vi "Main On Compile Action VI_Parse DMA Block Prop.vi"(5 "Decimation FIFO Index":i32, 8 "error in (no error)":errorcluster, 9 "FIFO indexes":i32[](array[numeric])=[1, 2, 3, 4, 5], 10 "Block Address":u32[](array[numeric])=[0, 2, 2, 0, 3], 11 "Relative Address in Block":u32[](array[numeric])=[0, 0, 1, 5, 5]) -> (0 "error out":errorcluster, 2 "Block descriptor":T1, 3 "max block size":u32)   [LabVIEW 2019, in "RefMem DMA System Explorer.lvlib"]
uses:
  RefMem DMA System Explorer.lvlib
  Shared/Block descriptor.ctl
  Shared/RefMem DMA Shared.lvlib
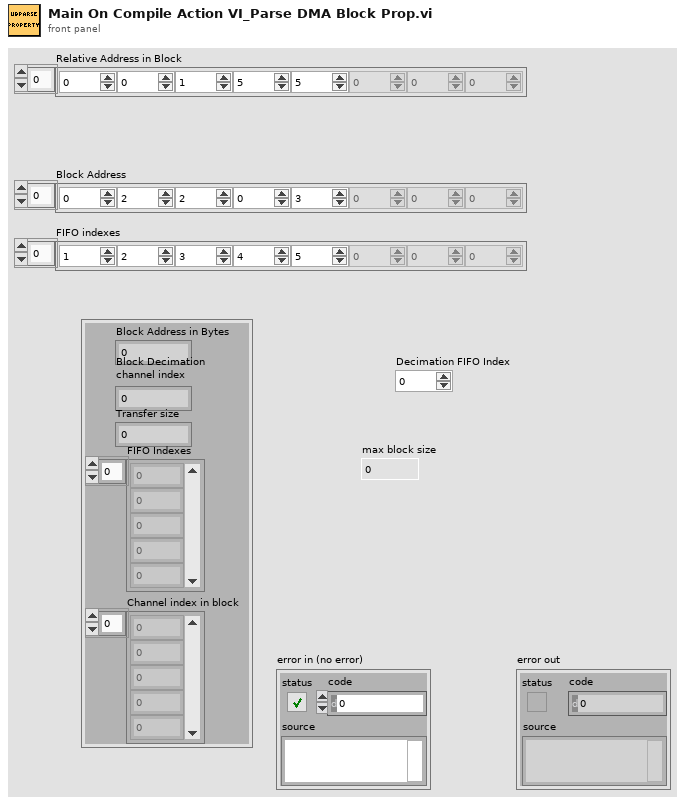
[diagram p1: front panel]
types:
  T1 = typedef "RefMem DMA Shared.lvlib/Block descriptor.ctl" = cluster{"Block Address in Bytes":u32, "Block Decimation \nchannel index":i32, "Transfer size":u32, "FIFO Indexes":i32[], "Channel index in block":i32[]}
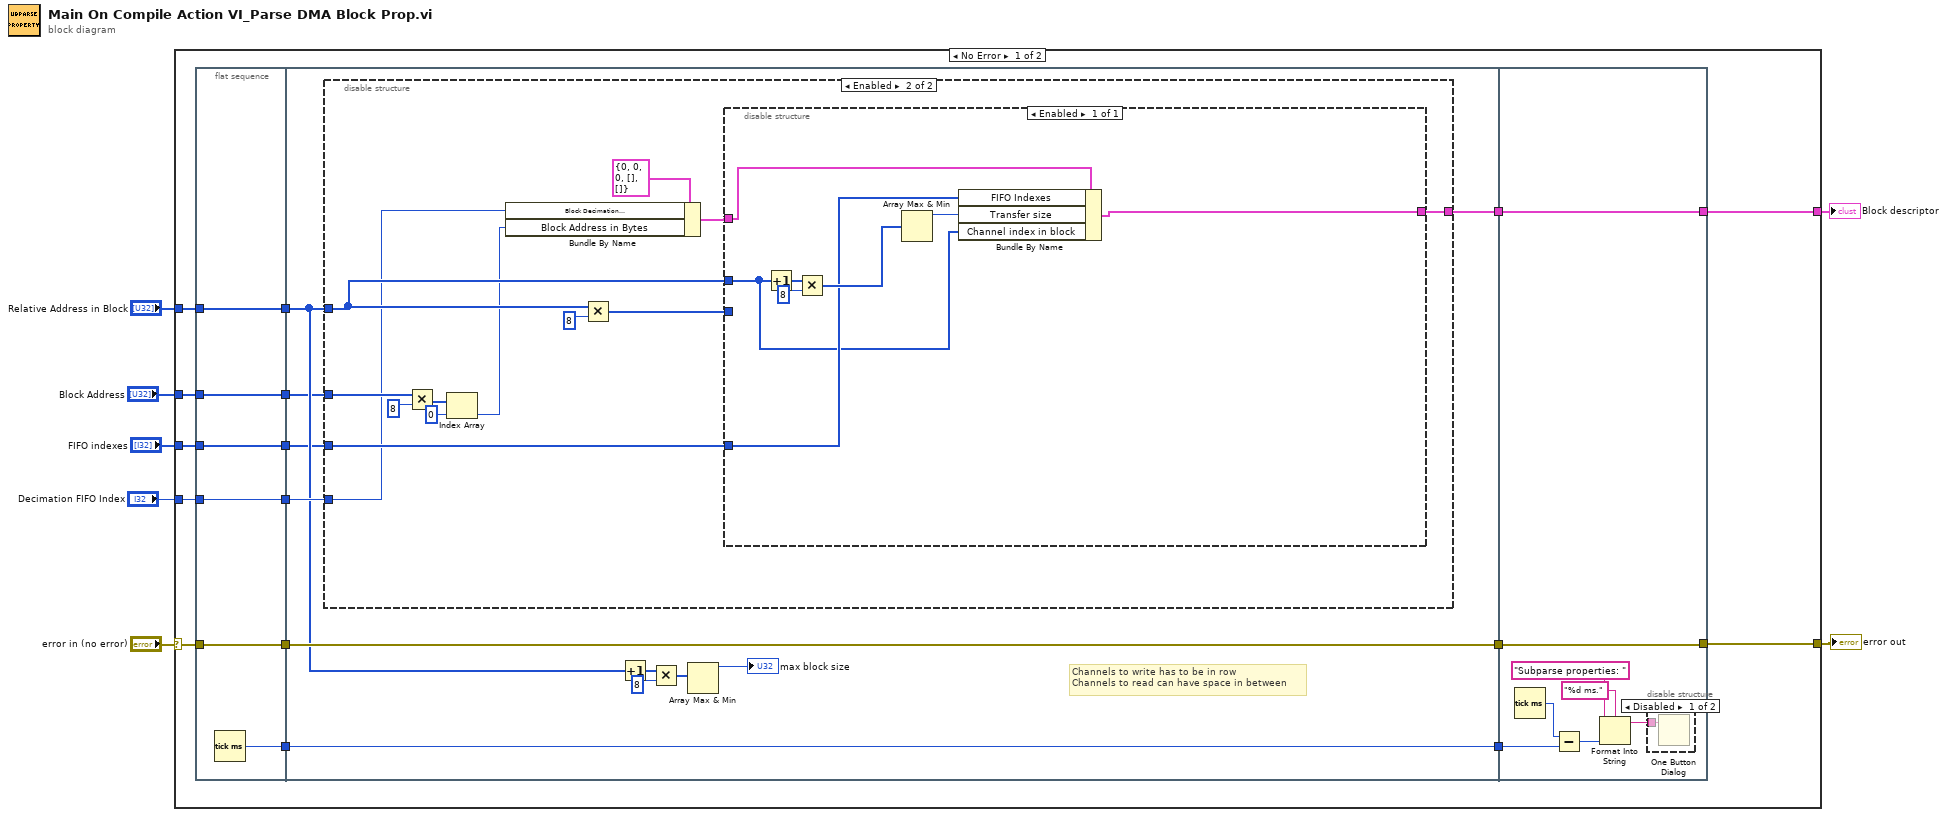
[diagram p0: block diagram]
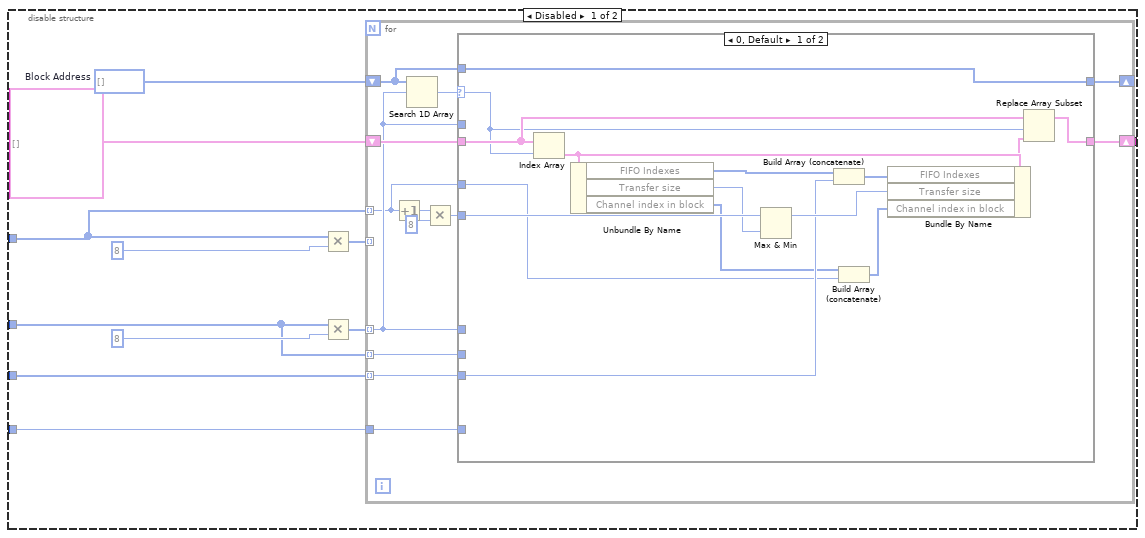
[diagram p2: hidden frame]
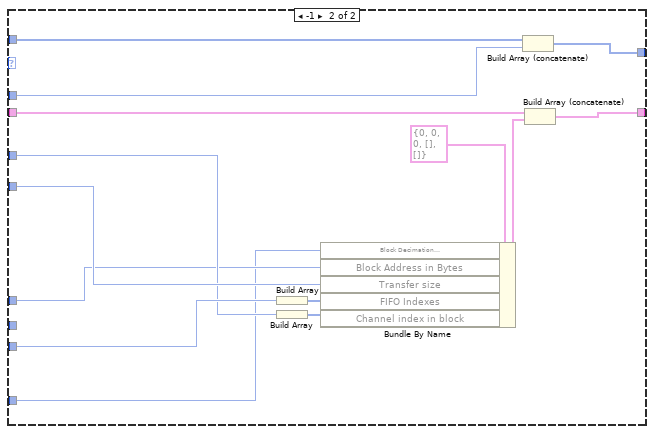
[diagram p3: hidden frame]
diagram:
  n1 = case shown="No Error" "error in (no error)" {
    selector: "error in (no error)" -> [w20 w124]
    tunnel: [w21 _] -> w7
    tunnel: [w18 w124] -> w5
    tunnel: "Decimation FIFO Index" -> [w17 _]
    tunnel: "Relative Address in Block" -> [w16 _]
    tunnel: "Block Address" -> [w15 _]
    tunnel: "FIFO indexes" -> [w14 _]
    frame No Error {
      n2 = flat-sequence {
        tunnel: w14 -> [w25]
        tunnel: w15 -> [w26]
        tunnel: w16 -> [w27]
        tunnel: w17 -> [w28]
        tunnel: w20 -> [w29]
        tunnel: [w29] -> w13
        tunnel: [w28] -> w12
        tunnel: [w27] -> w11
        tunnel: [w26] -> w10
        tunnel: [w25] -> w9
        tunnel: [w24] -> w8
        tunnel: [w40] -> w23
        tunnel: [w30] -> w22
        tunnel: [w35] -> w19
        tunnel: w13 -> [w35]
        tunnel: w12 -> [w34]
        tunnel: w11 -> [w33]
        tunnel: w10 -> [w32]
        tunnel: w9 -> [w31]
        tunnel: w8 -> [w30]
        tunnel: [w122] -> w21
        tunnel: w23 -> [w122]
        tunnel: w22 -> [w120]
        tunnel: w19 -> [w115]
        tunnel: [w115] -> w18
        frame #0 {
          n3 = Tick Count (ms)() -> (millisecond timer value=w24:u32)
        }
        frame #1 {
          # "Channels to write has to be in row\nChannels to read can have space in between"
          n4 = disable-structure shown="Enabled" {
            disable-tunnel: [w49 w106] -> w40
            disable-tunnel: w34 -> [w44 w98]
            disable-tunnel: w33 -> [w43 w102]
            disable-tunnel: w32 -> [w42 w101]
            disable-tunnel: w31 -> [w41 w100]
            frame Disabled {
              w51 = u32[] []  # Block Address
              n5 = Multiply(x=w43, y=u32 8) -> (x*y=w47:u32[])
              n6 = Multiply(x=w42, y=u32 8) -> (x*y=w45:u32[])
              n7 = for {
                tunnel: w45 -> [w59] mode=indexing
                tunnel: w41 -> [w58] mode=indexing
                shift-right: [w61] -> _
                shift-left: w51 -> [w63]
                shift-right: [w60] -> w49
                shift-left: T1[] [] ("Array out") -> [w62]
                tunnel: w47 -> [_] mode=indexing
                tunnel: w43 -> [w54] mode=indexing
                tunnel: w42 -> [w53] mode=indexing
                tunnel: w44 -> [w52]
                n8 = Increment(x=w54) -> (x+1=w57:u32)
                n9 = Search 1D Array(1D array=w63, element=w59) -> (index of element=w64:i32)  [unwired: 1 in]
                n10 = Multiply(x=w57, y=u32 8) -> (x*y=w55:u32)
                n11 = case shown="0, Default" w64 {
                  selector: w64 -> [w77 _]
                  tunnel: w63 -> [w74 w93]
                  tunnel: w62 -> [w78 w92]
                  tunnel: [w74 w91] -> w61
                  tunnel: [w76 w90] -> w60
                  tunnel: w59 -> [_ w89]
                  tunnel: w59 -> [_ w81]
                  tunnel: w58 -> [w68 w86]
                  tunnel: w55 -> [w73 w84]
                  tunnel: w54 -> [w65 w82]
                  tunnel: w52 -> [_ w80]
                  tunnel: w53 -> [_ _]
                  frame 0, Default {
                    n12 = Index Array(array=w78, index=w77) -> (element=w79:T1)
                    n13 = Unbundle By Name(w79) -> ("FIFO Indexes"=w70:i32[], "Transfer size"=w72:u32, "Channel index in block"=w66:i32[])
                    n14 = Max & Min(x=w73, y=w72) -> (max(x,y)=w71:u32)  [unwired: 1 out]
                    n15 = Build Array (concatenate)(w70, w68) -> (w69:i32[])
                    n16 = Build Array (concatenate)(w66, w65) -> (w67:u32[])
                    n17 = Bundle By Name(cluster=w79, "FIFO Indexes"=w69, "Transfer size"=w71, "Channel index in block"=w67) -> (w75:T1)
                    n18 = Replace Array Subset(array=w78, new element=w75, index=w77) -> (w76:T1[])
                  }
                  frame -1 {
                    n19 = Build Array(w86) -> (w85:i32[])
                    n20 = Build Array(w82) -> (w83:u32[])
                    n21 = Bundle By Name(cluster=T1 {"Block Address in Bytes"=0, "Block Decimation \nchannel index"=0, "Transfer size"=0, "FIFO Indexes"=[], "Channel index in block"=[]} ("Block descriptor"), "Block Decimation \nchannel index"=w80, "Block Address in Bytes"=w81, "Transfer size"=w84, "FIFO Indexes"=w85, "Channel index in block"=w83) -> (w87:T1)
                    n22 = Build Array (concatenate)(w93, w89) -> (w91:u32[])
                    n23 = Build Array (concatenate)(w92, w87) -> (w90:T1[])
                  }
                }
              }
            }
            frame Enabled {
              n24 = Multiply(x=w101, y=u32 8) -> (x*y=w96:u32[])
              n25 = Index Array(array=w96, index=0) -> (element=w95:u32)
              n26 = Bundle By Name(cluster=T1 {"Block Address in Bytes"=0, "Block Decimation \nchannel index"=0, "Transfer size"=0, "FIFO Indexes"=[], "Channel index in block"=[]} ("Block descriptor"), "Block Decimation \nchannel index"=w98, "Block Address in Bytes"=w95) -> (w97:T1)
              n27 = Multiply(x=w102, y=u32 8) -> (x*y=w104:u32[])
              n28 = disable-structure shown="Enabled" {
                disable-tunnel: [w114] -> w106
                disable-tunnel: w104 -> [_]
                disable-tunnel: w102 -> [w107]
                disable-tunnel: w100 -> [w108]
                disable-tunnel: w97 -> [w113]
                frame Enabled {
                  n29 = Increment(x=w107) -> (x+1=w112:u32[])
                  n30 = Multiply(x=w112, y=u32 8) -> (x*y=w110:u32[])
                  n31 = Array Max & Min(array=w110) -> (max value=w109:u32)  [unwired: 3 out]
                  n32 = Bundle By Name(cluster=w113, "FIFO Indexes"=w108, "Transfer size"=w109, "Channel index in block"=w107) -> (w114:T1)
                }
              }
            }
          }
          n33 = Increment(x=w33) -> (x+1=w37:u32[])
          n34 = Multiply(x=w37, y=u32 8) -> (x*y=w36:u32[])
          n35 = Array Max & Min(array=w36) -> (max value=→"max block size":u32)  [unwired: 3 out]
        }
        frame #2 {
          n36 = Tick Count (ms)() -> (millisecond timer value=w121:u32)
          n37 = Subtract(x=w121, y=w120) -> (x-y=w119:u32)
          n38 = Format Into String(format string="%d ms.", initial string="Subparse properties: ", w119) -> (resulting string=w116:string)  [unwired: 1 in, 1 out]
          n39 = disable-structure shown="Disabled" {
            disable-tunnel: w116 -> [w123 _]
            frame Disabled {
              n40 = One Button Dialog(message=w123) -> ()  [unwired: 1 in, 1 out]
            }
            frame Enabled {
            }
          }
        }
      }
    }
    frame Error {
    }
  }
  "Block descriptor" <- w7
  "error out" <- w5
